vi "Navigate Tree-Get Child.vi"(8 "error in (no error)":errorcluster, 10 "Tag":string, 11 "TreeControl in":refnum<class "TreeControl.lvclass">) -> (0 "error out":errorcluster, 2 "Navigate Tree:Get Child":string, 3 "TreeControl out":refnum<class "TreeControl.lvclass">)   [LabVIEW 2020, in "TreeControl.lvclass"]
doc: "Returns the tag of the first child item under an item. If the item has no child items, the method returns an empty string.\n\n Example\n\nQControl Class wrapper around the <b>TreeControl : Navigate Tree:Get Child Method</b>.\n<b> </b> <b> </b>\n©2016 Q Software Innovations, LLC (QSI)\nwritten by Quentin Alldredge\nproduced in LabVIEW 2015\n\nsupport@qsoftwareinnovations.com\nwww.qsoftwareinnovations.com\n\nAll rights reserved.\n\nRedistribution and use in source and binary forms, with or without modification, are permitted provided that the following conditions are met:\n\n * Redistributions of source code must retain the above copyright notice, this list of conditions and the following disclaimer.\n * Redistributions in binary form must reproduce the above copyright notice, this list of conditions and the following disclaimer in the documentation and/or other materials provided with the distribution.\n * Neither the name of Q Software Innovations, LLC. nor the names of its contributors may be used to endorse or promote products derived from this software without specific prior written permission.\n\nTHIS SOFTWARE IS PROVIDED BY THE COPYRIGHT HOLDERS AND CONTRIBUTORS \"AS IS\" AND ANY EXPRESS OR IMPLIED WARRANTIES, INCLUDING, BUT NOT LIMITED TO, THE IMPLIED WARRANTIES OF MERCHANTABILITY AND FITNESS FOR A PARTICULAR PURPOSE ARE DISCLAIMED. IN NO EVENT SHALL THE COPYRIGHT OWNER OR CONTRIBUTORS BE LIABLE FOR ANY DIRECT, INDIRECT, INCIDENTAL, SPECIAL, EXEMPLARY, OR CONSEQUENTIAL DAMAGES (INCLUDING, BUT NOT LIMITED TO, PROCUREMENT OF SUBSTITUTE GOODS OR SERVICES; LOSS OF USE, DATA, OR PROFITS; OR BUSINESS INTERRUPTION) HOWEVER CAUSED AND ON ANY THEORY OF LIABILITY, WHETHER IN CONTRACT, STRICT LIABILITY, OR TORT (INCLUDING NEGLIGENCE OR OTHERWISE) ARISING IN ANY WAY OUT OF THE USE OF THIS SOFTWARE, EVEN IF ADVISED OF THE POSSIBILITY OF SUCH DAMAGE."
uses:
  TreeControl.lvclass
  TreeControl.lvclass/TreeControl.ctl
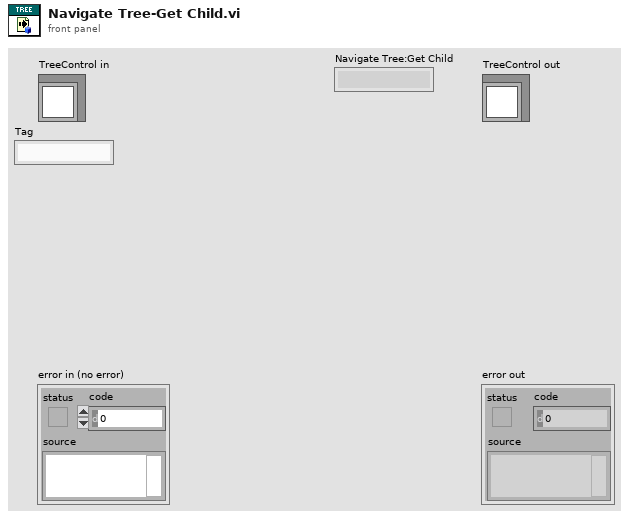
[diagram p1: front panel]
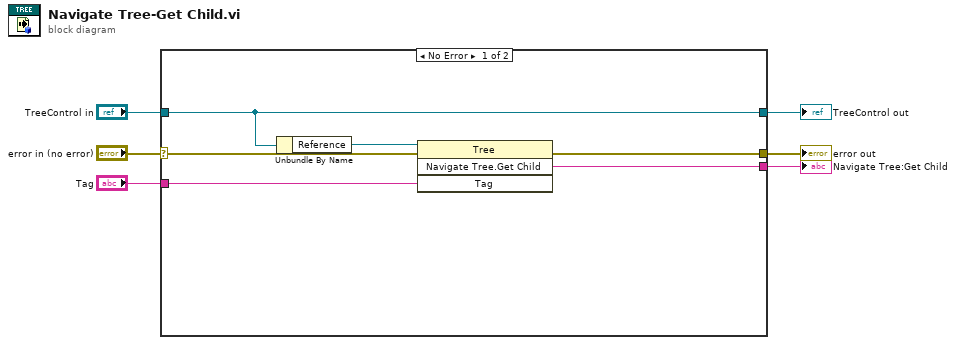
[diagram p0: block diagram]
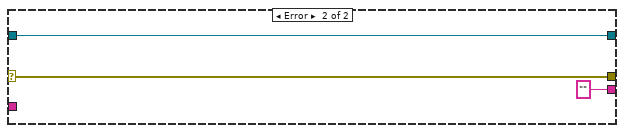
[diagram p2: hidden frame]
diagram:
  n1 = case shown="No Error" "error in (no error)" {
    selector: "error in (no error)" -> [w12 w15]
    tunnel: [w11 w15] -> w5
    tunnel: [w10 w14] -> w3
    tunnel: "TreeControl in" -> [w10 w14]
    tunnel: "Tag" -> [w8 _]
    tunnel: [w7 "" ("Navigate Tree:Get Child")] -> w1
    frame No Error {
      n2 = Unbundle By Name(w10) -> ("Reference"=w9:refnum<vi>)
      n3 = invoke class="Tree" method="Navigate Tree.Get Child"(reference=w9, error in=w12, "Tag"=w8) -> (error out=w11:errorcluster, "Navigate Tree:Get Child"=w7:string)  [unwired: 1 in, 2 out]
    }
    frame Error {
    }
  }
  "error out" <- w5
  "TreeControl out" <- w3
  "Navigate Tree:Get Child" <- w1
